vi "automated_scan_v1.0.vi"() -> ()   [LabVIEW 2018]
uses:
  Other Libraries/MoCo Software/VI/global_m.vi
  <vilib>/Utility/file.llb/Write Delimited Spreadsheet (DBL).vi
  <vilib>/Utility/file.llb/Write Delimited Spreadsheet (string).vi
  Other Libraries/Thorlabs_FW102C/Thorlabs_FW102C.lvlib
panel:
  out "nloops":i32
  out "FW Position":i32
  out "Filter Wheel":errorcluster
  out "Current Wavelength(nm)":dbl
  out "Take Image":errorcluster
  out "Dark Integrating Time (s)":dbl caption="Elapsed Time (s)"
  out "% complete":dbl
  out "Total Steps":dbl
  in  "Tab Control":T1(tab)
  in  "Photodiode (VISA resource name)[Com3]":refnum<visa-resource-name>="COM3"
  in  "Mono port":refnum<visa-resource-name>="COM2"
  in  "Grating, gr/mm":u16(ring)=2 items=["2400", "1800", "1200", "600", "300", "150"]
  in  "Take Image":bool=TRUE
  in  "Step Size":dbl=10.0
  in  "Stop Wavelength":dbl=600.0
  in  "Start Wavelength":dbl=500.0
  in  "Scan Directory":string="Peter_ferguson\\Tcal\\scans\\"
  in  "Scan Name":string="test_scan"
  in  "Scan Type":string(combo)="New Scan"
  in  "Photodiode / Camera\n Integration time(s)":dbl=10.0
  in  "Spectrometer Integration time":dbl=0.001
  out "VISA out":refnum<visa-resource-name>
  out "Current Value Bin":dbl format="%.6f"
  out "dup VISA session":refnum<visa-resource-name>
  out "dup VISA session 2":refnum<visa-resource-name>
  out "Mono wav":dbl format="%.3f"
  out "Photodiode 2":errorcluster
  out "Light Integrating Time (s)":dbl caption="Elapsed Time (s)"
  out "Active Wavelength":u32
  out "Serial Number":string
  out "Mono/Photodiode":errorcluster
  out "Step #":i32
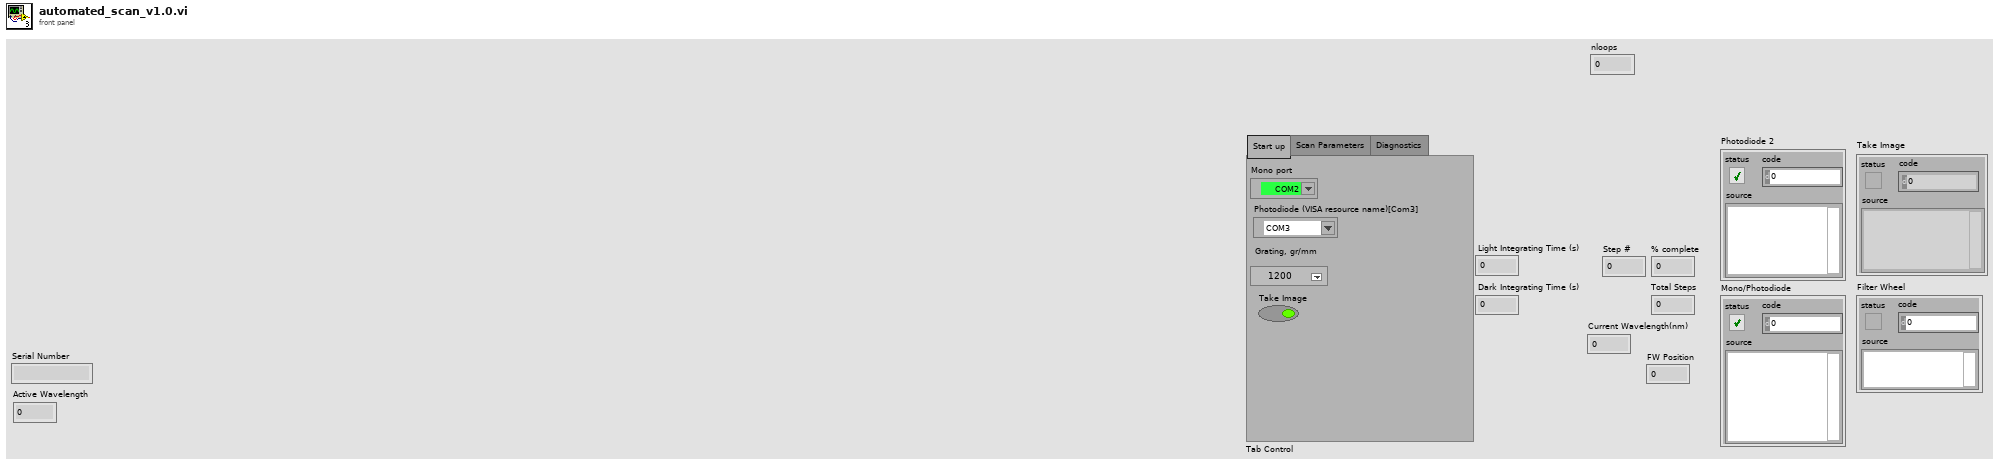
[diagram p1: front panel]
types:
  T1 = enum32{"Start up", "Scan Parameters", "Diagnostics"}
  T2 = cluster{"Head Type":u32, "Head Version":u32, "Serial Number":string, "Calibration Sensitivity":dbl, "Default Wavelength":u32, "Active Sensitivity":dbl, "Active Wavelength":u32, "Scale Min Power (Wattmeter)":u32, "Scale Max Power (Wattmeter)":u32, "Scale Min Energy":u32, "Scale Max Energy":u32, "Current Scale":u32, "Calo Mode":bool, "Anticipation":bool, "External Trig":bool, "Trig Level":dbl, "Zero Offset":dbl, "Multiplier 1":dbl, "Offset 1":dbl, "Multiplier 2":dbl, "Offset 2":dbl, "Max Power (Joulemeter)":dbl, "Max energy (Joulemeter)":dbl, "Currently Logging":bool, "Analog Out Active":bool, "Resolution":dbl, "Currently Calculating Stats":bool, "High-Resolution Display":bool, "Scale Min Wavelenght":u32, "Scale Max Wavelenght":u32, "Upper Bound":dbl, "Lower Bond":dbl, "Reference Value":dbl, "Thresholds Active":bool, "Fail":bool, "Attenuator":bool, "autoScale":bool, "IsdBm":bool}
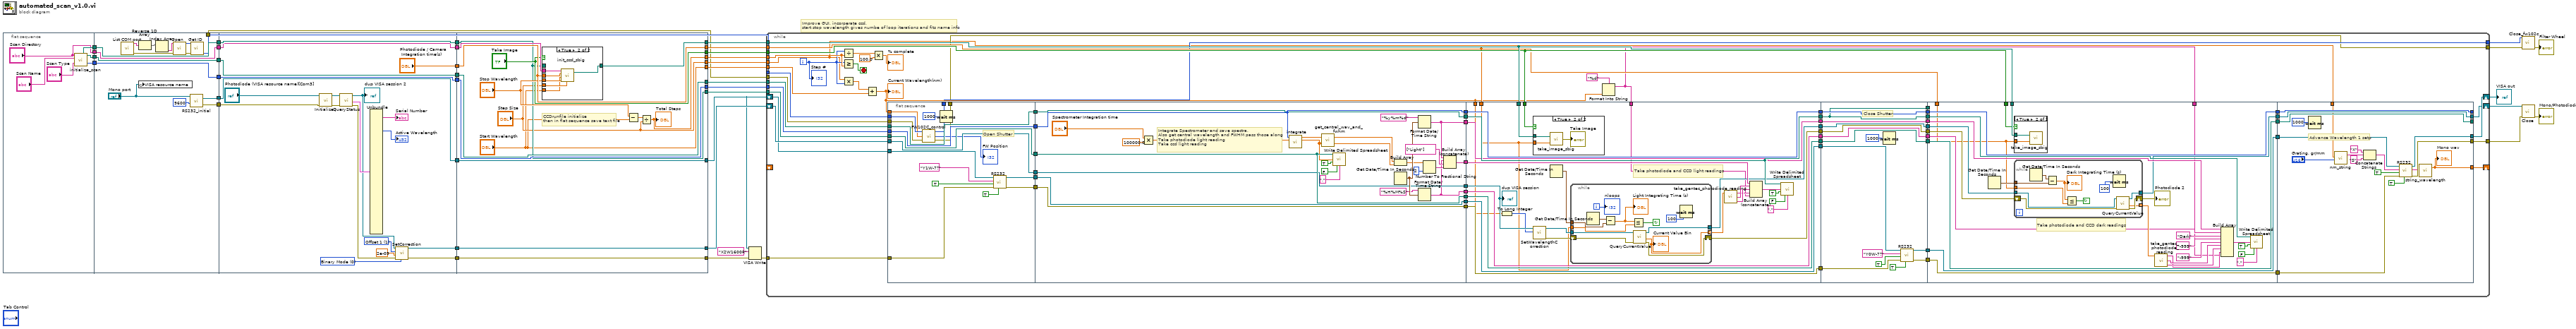
[diagram p0: block diagram]
diagram:
  # "Improve GUI, incorperate ccd,\nstart stop wavelength gives numbe of loop iterations and fits name info"
  n1 = flat-sequence {
    tunnel: [w45] -> w29
    tunnel: [w44] -> w28
    tunnel: [w43] -> w27
    tunnel: ["Scan Directory"] -> w13
    tunnel: [w61] -> w26
    tunnel: [w60] -> w25
    tunnel: w29 -> [w59]
    tunnel: [w59] -> w24
    tunnel: w28 -> [w58]
    tunnel: [w58] -> w23
    tunnel: w27 -> [w57]
    tunnel: [w57] -> w22
    tunnel: w13 -> [w56]
    tunnel: [w56] -> w11
    tunnel: [w49] -> w5
    tunnel: [w48] -> w4
    tunnel: w26 -> [w76]
    tunnel: [w76] -> w21
    tunnel: w25 -> [w72]
    tunnel: w24 -> [w75]
    tunnel: [w75] -> w20
    tunnel: w23 -> [w74]
    tunnel: [w74] -> w19
    tunnel: w22 -> [w73]
    tunnel: [w73] -> w18
    tunnel: [w69] -> w17
    tunnel: ["Photodiode / Camera\n Integration time(s)"] -> w16
    tunnel: [w65] -> w15
    tunnel: [w71] -> w12
    tunnel: w11 -> [w71]
    tunnel: [w96] -> w31
    tunnel: w21 -> [w96]
    tunnel: [w86] -> w39
    tunnel: w20 -> [w86]
    tunnel: [w95] -> w38
    tunnel: w19 -> [w95]
    tunnel: [w94] -> w37
    tunnel: w18 -> [w94]
    tunnel: [w93] -> w36
    tunnel: w17 -> [w93]
    tunnel: [w90] -> w35
    tunnel: w16 -> [w90]
    tunnel: [w97] -> w30
    tunnel: w15 -> [w92]
    tunnel: [w92] -> w14
    tunnel: w12 -> [w91]
    tunnel: [w88] -> w10
    tunnel: ["Take Image"] -> w9
    tunnel: ["Step Size"] -> w7
    tunnel: ["Start Wavelength"] -> w6
    frame #0 {
      n2 = call "initialize_scan.vi"("Scan Directory"="Scan Directory", "Scan Name"="Scan Name", "Scan Type"="Scan Type") -> ("Path Spec"=w45:path, "Path Scan"=w43:path, "Wrapper Out"=w44:u64)  [unwired: 8 in, 2 out]
    }
    frame #1 {
      n3 = call "List COM port.vi"() -> ("error out"=w50:errorcluster, "COM Ports"=w53:string[])  [unwired: 10 in]
      n4 = Reverse 1D Array(array=w53) -> (reversed array=w52:string[])
      n5 = global write "global_m.vi" "VISA resource name"("Mono port") -> ()
      n6 = Index Array(array=w52) -> (element=w51:string)  [unwired: 1 in]
      n7 = call "Open.vi"("error in (no error)"=w50, "Serial Port"=w51) -> ("error out"=w54:errorcluster, "FW102C out"=w55:i32)  [unwired: 7 in, 1 out]
      n8 = call "RS232_initial.vi"("baud rate"=u32 9600, "VISA resource name"="Mono port") -> ("error out"=w60:errorcluster, "VISA name out"=w61:refnum<visa-resource-name>)  [unwired: 2 in]
      n9 = call "Get ID.vi"("error in (no error)"=w54, "FW102C in"=w55) -> ("error out"=w48:errorcluster, "FW102C out"=w49:i32)  [unwired: 7 in, 1 out]
    }
    frame #2 {
      w64 = u16 0 items=["Binary Mode", "Text Mode"] ("Transfer Type (binary)")
      w68 = u16 1 items=["Multiplier1", "Offset 1", "Multiplier 2", "Offset 2"] ("Correction Type")
      n10 = call "Initialize2.vi"("error in (no error)"=w72, "Instr. Descriptor (GPIB::)"="Photodiode (VISA resource name)[Com3]") -> ("error out"=w78:errorcluster, "VISA session"=w82:refnum<visa-resource-name>)  [unwired: 4 in]
      n11 = call "QueryStatus.vi"("error in (no error)"=w78, "VISA session"=w82) -> ("error out"=w66:errorcluster, "Status Data"=w81:T2, "dup VISA session"=w70:refnum<visa-resource-name>)  [unwired: 4 in, 1 out]
      "dup VISA session 2" <- w70
      n12 = Unbundle(w81) -> ("Serial Number"=→"Serial Number":string, "Active Wavelength"=→"Active Wavelength":u32)  [unwired: 36 out]
      n13 = call "SetCorrection.vi"("Transfer Type (binary)"=w64, "error in (no error)"=w66, "Correction  Value"=2e-09, "Correction Type"=w68, "VISA session"=w70) -> ("error out"=w65:errorcluster, "dup VISA session"=w69:refnum<visa-resource-name>)  [unwired: 3 in]
    }
    frame #3 {
      # "CCDrunfile initialize\nthen in flat sequence save text file"
      n14 = case shown="True" "Take Image" {
        tunnel: w91 -> [_ w105]
        tunnel: w90 -> [_ w104]
        tunnel: "Step Size" -> [_ w103]
        tunnel: "Stop Wavelength" -> [_ w102]
        tunnel: [w99 w101] -> w88
        tunnel: "Start Wavelength" -> [_ w100]
        tunnel: w86 -> [w99 _]
        frame False {
        }
        frame True {
          n15 = call "init_ccd_sbig.vi"("Scan Directory"=w105, "Exposure Time"=w104, "Min nm"=w100, "Max nm"=w102, "Step size"=w103) -> ("Working Directory"=w101:path)  [unwired: 1 in]
        }
      }
      n16 = Subtract(x="Stop Wavelength", y="Start Wavelength") -> (x-y=w98:dbl)
      n17 = Divide(x=w98, y="Step Size") -> (x/y=w97:dbl)
      "Total Steps" <- w97
    }
  }
  n18 = VISA Write(VISA resource name=w31, write buffer="X2W1600R", error in (no error)=w14) -> (error out=w40:errorcluster)  [unwired: 2 out]
  n19 = while {
    tunnel: w40 -> [w173]
    tunnel: [w172] -> w34
    tunnel: w39 -> [w171]
    tunnel: w38 -> [w170]
    shift-right: [w124] -> _
    shift-left: _ -> [_]
    tunnel: w37 -> [w157]
    tunnel: w35 -> [w114]
    shift-right: [w125] -> w8
    shift-left: w36 -> [w147]
    shift-right: [w128] -> w32
    shift-left: w31 -> [w126]
    tunnel: w30 -> [w123]
    tunnel: w10 -> [w119]
    tunnel: w9 -> [w118]
    tunnel: w7 -> [w106]
    tunnel: w6 -> [w117]
    tunnel: w5 -> [w112]
    tunnel: w4 -> [w111]
    tunnel: [w109] -> w1
    tunnel: [w108] -> w2
    i -> [w115]
    stop <- w136 stop-if-true
    n20 = Divide(x=w115, y=w123) -> (x/y=w122:dbl)
    n21 = Greater Or Equal?(x=w115, y=w123) -> (x >= y?=w136:bool)
    n22 = Multiply(x=w106, y=w115) -> (x*y=w116:dbl)
    n23 = Add(x=w116, y=w117) -> (x+y=w110:dbl)
    "Current Wavelength(nm)" <- w110
    n24 = Multiply(x=w122, y=100.0) -> (x*y=→"% complete":dbl)
    n25 = flat-sequence {
      tunnel: w173 -> [w190]
      tunnel: [w189] -> w169
      tunnel: [w188] -> w168
      tunnel: [w184] -> w167
      tunnel: w171 -> [w184]
      tunnel: w170 -> [w183]
      tunnel: [w183] -> w166
      tunnel: w157 -> [w182]
      tunnel: [w182] -> w156
      tunnel: w147 -> [w181]
      tunnel: [w181] -> w146
      tunnel: w126 -> [w180]
      tunnel: w112 -> [w179]
      tunnel: w111 -> [w178]
      tunnel: w110 -> [w177]
      tunnel: [w176] -> w109
      tunnel: [w175] -> w108
      tunnel: w169 -> [w217]
      tunnel: [w217] -> w155
      tunnel: w168 -> [w216]
      tunnel: [w216] -> w154
      tunnel: w167 -> [w208]
      tunnel: [w208] -> w153
      tunnel: w166 -> [w209]
      tunnel: [w209] -> w151
      tunnel: w156 -> [w197]
      tunnel: [w197] -> w149
      tunnel: [w196] -> w148
      tunnel: w146 -> [w195]
      tunnel: [w195] -> w145
      tunnel: [w193] -> w135
      tunnel: [w192] -> w130
      tunnel: w155 -> [w243]
      tunnel: w154 -> [w230]
      tunnel: w153 -> [w245]
      tunnel: [w245] -> w152
      tunnel: w151 -> [w244]
      tunnel: [w244] -> w150
      tunnel: w149 -> [w229]
      tunnel: w148 -> [w234]
      tunnel: w145 -> [w242]
      tunnel: [w243] -> w144
      tunnel: w114 -> [w222]
      tunnel: [w230] -> w143
      tunnel: [w229] -> w142
      tunnel: [w228] -> w140
      tunnel: [w227] -> w137
      tunnel: w135 -> [w226]
      tunnel: [w226] -> w134
      tunnel: [w225] -> w131
      tunnel: w130 -> [w225]
      tunnel: w119 -> [w223]
      tunnel: w118 -> [w221]
      tunnel: w107 -> [w218]
      tunnel: w110 -> [w220]
      tunnel: [w274] -> w165
      tunnel: [w273] -> w163
      tunnel: w152 -> [w269]
      tunnel: [w269] -> w161
      tunnel: [w268] -> w159
      tunnel: w150 -> [w268]
      tunnel: w144 -> [w267]
      tunnel: w143 -> [w266]
      tunnel: w142 -> [w261]
      tunnel: [w261] -> w141
      tunnel: w140 -> [w265]
      tunnel: [w265] -> w139
      tunnel: [w264] -> w138
      tunnel: w137 -> [w264]
      tunnel: w134 -> [w263]
      tunnel: [w263] -> w133
      tunnel: [w262] -> w132
      tunnel: w131 -> [w262]
      tunnel: [w261] -> w129
      tunnel: w165 -> [w302]
      tunnel: [w302] -> w164
      tunnel: w163 -> [w301]
      tunnel: [w301] -> w162
      tunnel: w161 -> [w300]
      tunnel: [w300] -> w160
      tunnel: w159 -> [w299]
      tunnel: [w299] -> w158
      tunnel: w141 -> [_]
      tunnel: w139 -> [w284]
      tunnel: w138 -> [w283]
      tunnel: w114 -> [w280]
      tunnel: w133 -> [w291]
      tunnel: w132 -> [w290]
      tunnel: w129 -> [w289]
      tunnel: [w282] -> w127
      tunnel: w119 -> [w279]
      tunnel: w118 -> [w278]
      tunnel: w107 -> [w276]
      tunnel: w164 -> [w330]
      tunnel: w162 -> [w331]
      tunnel: w160 -> [w320]
      tunnel: w158 -> [w322]
      tunnel: [w329] -> w128
      tunnel: [w328] -> w172
      tunnel: [w322] -> _
      tunnel: [w320] -> _
      tunnel: [w319] -> w125
      tunnel: w127 -> [w319]
      tunnel: [w318] -> w124
      tunnel: w106 -> [w317]
      frame #0 {
        # "Open Shutter"
        n26 = call "FW102C_control.vi"("error in (no error)"=w178, "Current Wavelength"=w177, "FW102C in"=w179) -> ("error out"=w175:errorcluster, "Position"=→"FW Position":i32, "FW102C out"=w176:i32)
        n27 = Wait (ms)(milliseconds to wait=u32 1000) -> ()  [unwired: 1 out]
        n28 = call "RS232.vi"("read"=TRUE, "error in"=w190, "write"=TRUE, "string to write"="Y1W-7?" ("string"), "VISA  name in"=w180) -> ("error out"=w188:errorcluster, "VISA out"=w189:refnum<visa-resource-name>)  [unwired: 1 in, 2 out]
      }
      frame #1 {
        # "Integrate Spectrometer and save spectra, \nAlso get central wavelength and FWHM pass those along\nTake photodiode light reading \nTake ccd light reading"
        n29 = Multiply(x="Spectrometer Integration time", y=100000.0) -> (x*y=w213:dbl)
        n30 = call "integrate.vi"("Numeric"=w213, "Wrapper Out"=w209) -> ("Spectrum Values"=w206:dbl[], "WL Values"=w207:dbl[])  [unwired: 7 in, 1 out]
        n31 = call "get_central_wav_and_fwhm.vi"("Signal"=w206, "Wavelenghs"=w207) -> ("FWHM"=w202:dbl, "Central"=w194:dbl)
        n32 = call-poly <vilib>:"Write Delimited Spreadsheet.vi"("file path (dialog if empty)"=w208, "1D data"=w206, "append to file? (new file:F)"=TRUE, "transpose? (no:F)"=FALSE, "delimiter (\\t)"="," ("delimiter (\\t)")) -> ()  [unwired: 9 in, 2 out]
        n33 = Build Array(w194, w202) -> (w201:dbl[])
        n34 = Get Date/Time In Seconds() -> (seconds since 1Jan1904=w204:timestamp)
        n35 = Format Date/Time String(time format string (%c)="%y%m%d", seconds (now)=w204) -> (date/time string=w193:string)  [unwired: 1 in]
        n36 = Format Date/Time String(time format string (%c)="%H%M%S", seconds (now)=w204) -> (date/time string=w192:string)  [unwired: 1 in]
        n37 = Number To Fractional String(number=w201, precision (6)=i16 2) -> (F-format string=w198:string[])  [unwired: 2 in]
        n38 = Build Array (concatenate)(w193, w192, string[] ["Light"] ("array"), w198) -> (w196:string[])
      }
      frame #2 {
        # "Take photodiode and CCD light readings"
        n39 = To Long Integer(number=w220) -> (32bit integer=w241:i32)
        n40 = case shown="True" w221 {
          tunnel: w223 -> [_ w248]
          tunnel: w222 -> [_ w247]
          frame False {
          }
          frame True {
            n41 = call "take_image_sbig.vi"("Exptime"=w247, "path"=w248) -> ("error out"=→"Take Image":errorcluster)
          }
        }
        n42 = call "SetWavelengthCorrection.vi"("Wave Length  ( 0= restore default)"=w241, "VISA session"=w242) -> ("error out"=w239:errorcluster, "dup VISA session"=w240:refnum<visa-resource-name>)  [unwired: 6 in]
        n43 = Get Date/Time In Seconds() -> (seconds since 1Jan1904=w224:timestamp)
        n44 = while {
          tunnel: w240 -> [w260]
          shift-right: [w258] -> w227
          shift-left: w239 -> [w259]
          tunnel: w222 -> [w256]
          tunnel: [w255] -> w235 mode=indexing
          tunnel: [w254] -> w228
          tunnel: w224 -> [w252]
          i -> [w250]
          stop <- w257 continue-if-true
          n45 = Get Date/Time In Seconds() -> (seconds since 1Jan1904=w253:timestamp)
          n46 = Subtract(x=w253, y=w252) -> (x-y=w251:dbl)
          "Light Integrating Time (s)" <- w251
          n47 = Less Or Equal?(x=w251, y=w256) -> (x <= y?=w257:bool)
          n48 = call "QueryCurrentValue.vi"("error in (no error)"=w259, "VISA session"=w260) -> ("error out"=w258:errorcluster, "Current Value Bin"=w255:dbl, "dup VISA session"=w254:refnum<visa-resource-name>)  [unwired: 3 in, 2 out]
          "Current Value Bin" <- w255
          n49 = Wait (ms)(milliseconds to wait=u32 100) -> ()  [unwired: 1 out]
          "nloops" <- w250
        }
        n50 = call "take_gentec_photodiode_reading.vi"("numeric array"=w235) -> ("SD"=w232:string, "Mean"=w233:string, "Num of readings"=w219:string)  [unwired: 2 in]
        n51 = Build Array (concatenate)(w234, w233, w232, w219, w218) -> (w231:string[])
        n52 = call-poly <vilib>:"Write Delimited Spreadsheet.vi"("file path (dialog if empty)"=w229, "1D data"=w231, "append to file? (new file:F)"=TRUE, "transpose? (no:F)"=FALSE, "delimiter (\\t)"="," ("delimiter (\\t)")) -> ()  [unwired: 9 in, 2 out]
        "dup VISA session" <- w242
      }
      frame #3 {
        # "Close Shutter"
        n53 = Wait (ms)(milliseconds to wait=u32 1000) -> ()  [unwired: 1 out]
        n54 = call "RS232.vi"("read"=TRUE, "error in"=w266, "write"=TRUE, "string to write"="Y0W-7?" ("string"), "VISA  name in"=w267) -> ("error out"=w273:errorcluster, "VISA out"=w274:refnum<visa-resource-name>)  [unwired: 1 in, 2 out]
      }
      frame #4 {
        # "Take photodiode and CCD dark readings"
        n55 = Get Date/Time In Seconds() -> (seconds since 1Jan1904=w281:timestamp)
        n56 = case shown="True" w278 {
          tunnel: w280 -> [_ w304]
          tunnel: w279 -> [_ w303]
          frame False {
          }
          frame True {
            n57 = call "take_image_sbig.vi"("Exptime"=w304, "path"=w303) -> ()  [unwired: 1 out]
          }
        }
        n58 = while {
          shift-right: [w314] -> w294
          shift-left: w283 -> [w315]
          tunnel: [w312] -> w295 mode=indexing
          tunnel: w280 -> [w311]
          tunnel: w284 -> [w310]
          tunnel: [w309] -> w282
          tunnel: w281 -> [w307]
          stop <- w313 continue-if-true
          n59 = Get Date/Time In Seconds() -> (seconds since 1Jan1904=w308:timestamp)
          n60 = Subtract(x=w308, y=w307) -> (x-y=w306:dbl)
          "Dark Integrating Time (s)" <- w306
          n61 = Less Or Equal?(x=w306, y=w311) -> (x <= y?=w313:bool)
          n62 = Wait (ms)(milliseconds to wait=u32 100) -> ()  [unwired: 1 out]
          n63 = call "QueryCurrentValue.vi"("error in (no error)"=w315, "VISA session"=w310) -> ("error out"=w314:errorcluster, "Current Value Bin"=w312:dbl, "dup VISA session"=w309:refnum<visa-resource-name>)  [unwired: 3 in, 2 out]
        }
        "Photodiode 2" <- w294
        n64 = call "take_gentec_photodiode_reading.vi"("numeric array"=w295) -> ("SD"=w288:string, "Mean"=w287:string, "Num of readings"=w277:string)  [unwired: 2 in]
        n65 = Build Array(w291, w290, "Dark" ("date/time string"), "-999" ("element"), "-999" ("element"), w287, w288, w277, w276) -> (w292:string[])
        n66 = call-poly <vilib>:"Write Delimited Spreadsheet.vi"("file path (dialog if empty)"=w289, "1D data"=w292, "append to file? (new file:F)"=TRUE, "transpose? (no:F)"=FALSE, "delimiter (\\t)"="," ("delimiter (\\t)")) -> ()  [unwired: 9 in, 2 out]
      }
      frame #5 {
        # "Advance Wavelength 1 setp"
        n67 = Wait (ms)(milliseconds to wait=u32 1000) -> ()  [unwired: 1 out]
        n68 = call "nm_string.vi"("Grating, gr/mm"="Grating, gr/mm", "Wavelength, nm"=w317) -> ("nm_String"=w327:string)  [unwired: 2 in, 1 out]
        n69 = Concatenate Strings("X" ("string"), w327, "S" ("string")) -> (w324:string)
        n70 = call "RS232.vi"("read"=TRUE, "error in"=w331, "write"=TRUE, "string to write"=w324, "VISA  name in"=w330) -> ("error out"=w328:errorcluster, "read string"=w321:string, "VISA out"=w329:refnum<visa-resource-name>)  [unwired: 1 in, 1 out]
        n71 = call "string_wavelength.vi"("Position String"=w321) -> ("Present Wavelength"=w318:dbl)  [unwired: 3 in, 1 out]
        "Mono wav" <- w318
      }
    }
    n72 = Format Into String(format string="%d", w110) -> (resulting string=w107:string)  [unwired: 2 in, 1 out]
    "Step #" <- w115
  }
  "VISA out" <- w32
  n73 = call "Close_fw102c.vi"("error in (no error)"=w2, "FW102C in"=w1) -> ("error out"=→"Filter Wheel":errorcluster)  [unwired: 9 in]
  n74 = call "Close.vi"("VISA session"=w8, "error in (no error)"=w34) -> ("error out"=→"Mono/Photodiode":errorcluster)  [unwired: 13 in]
